vi "acquire single wave by LAN init subvi.vi"(0 "TCP Network Connection in":refnum<k5>, 11 "error in (no error)":errorcluster) -> (1 "CH1":string, 2 "Array 3":string[](array[string]), 3 "SEC/DIV":string, 4 "TCP Network Connection out":refnum<k5>, 6 "Array 2":string[](array[string]), 8 "Numeric":i32, 10 "data out":string, 13 "ID Query":string, 14 "Array":string[](array[string]), 15 "error out":errorcluster)   [LabVIEW 2013]
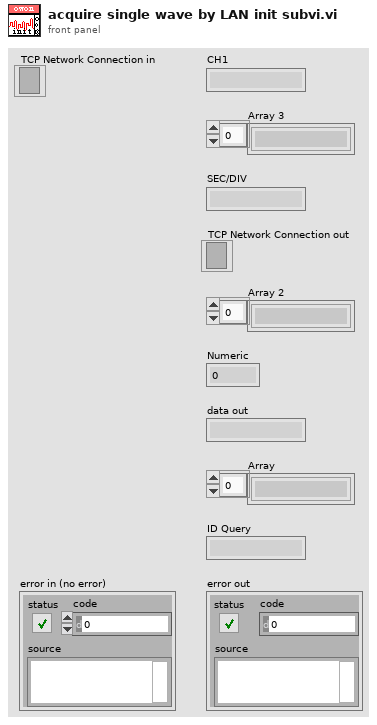
[diagram p1: front panel]
types:
  T1 = enum16{"Standard", "Buffered", "CRLF", "Immediate"}
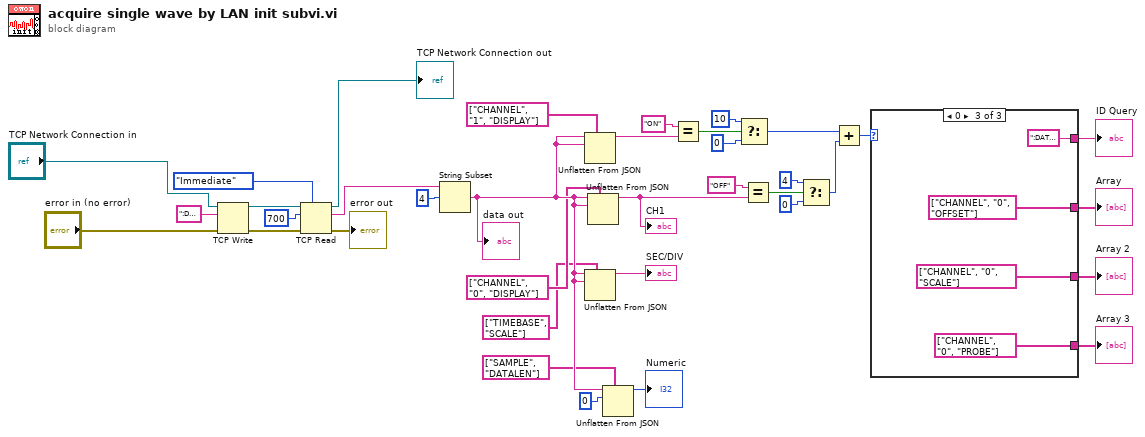
[diagram p0: block diagram]
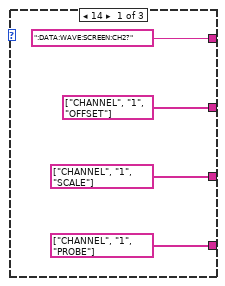
[diagram p2: hidden frame]
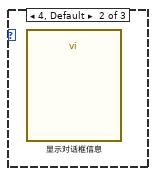
[diagram p3: hidden frame]
diagram:
  n1 = TCP Write(connection ID="TCP Network Connection in", data in=":DATA:WAVE:SCREEN:HEAD?" ("ID Query"), error in (no error)="error in (no error)") -> (connection ID out=w6:refnum<k5>, error out=w7:errorcluster)  [unwired: 1 in, 1 out]
  n2 = TCP Read(connection ID=w6, bytes to read=u32 700 ("byte count"), error in (no error)=w7, 7:T1."Immediate" ("mode (standard)")) -> (connection ID out=→"TCP Network Connection out":refnum<k5>, data out=w10:string, error out=→"error out":errorcluster)  [unwired: 1 in]
  n3 = String Subset(string=w10, offset (0)=4) -> (substring=w36:string)  [unwired: 1 in]
  "data out" <- w36
  n4 = Unflatten From JSON(path=string[] ["CHANNEL", "1", "DISPLAY"], JSON string=w36, type and defaults=w36) -> (value=w23:string)  [unwired: 4 in, 1 out]
  n5 = Unflatten From JSON(path=string[] ["TIMEBASE", "SCALE"], JSON string=w36, type and defaults=w36) -> (value=→"SEC/DIV":string)  [unwired: 4 in, 1 out]
  n6 = Unflatten From JSON(path=string[] ["CHANNEL", "0", "DISPLAY"], JSON string=w36, type and defaults=w36) -> (value=w29:string)  [unwired: 4 in, 1 out]
  "CH1" <- w29
  n7 = Unflatten From JSON(path=string[] ["SAMPLE", "DATALEN"], JSON string=w36, type and defaults=0) -> (value=→"Numeric":i32)  [unwired: 4 in, 1 out]
  n8 = Equal?(x="ON", y=w23) -> (x = y?=w25:bool)
  n9 = Select(t=10 ("offset (0)"), s=w25, f=0 ("offset (0)")) -> (s? t:f=w33:i32)
  n10 = Equal?(x="OFF", y=w29) -> (x = y?=w32:bool)
  n11 = Select(t=4 ("offset (0)"), s=w32, f=0 ("offset (0)")) -> (s? t:f=w34:i32)
  n12 = Add(x=w33, y=w34) -> (x+y=w35:i32)
  n13 = case shown="0" w35 {
    tunnel: [":DATA:WAVE:SCREEN:CH2?" ("ID Query") _ ":DATA:WAVE:SCREEN:CH1?" ("ID Query")] -> w19
    tunnel: [string[] ["CHANNEL", "1", "PROBE"] _ string[] ["CHANNEL", "0", "PROBE"]] -> w13
    tunnel: [string[] ["CHANNEL", "1", "SCALE"] _ string[] ["CHANNEL", "0", "SCALE"]] -> w14
    tunnel: [string[] ["CHANNEL", "1", "OFFSET"] _ string[] ["CHANNEL", "0", "OFFSET"]] -> w15
    frame 14 {
    }
    frame 4, Default {
      n14 = call "显示对话框信息"() -> ()  [unwired: 10 in, 2 out]
    }
    frame 0 {
    }
  }
  "ID Query" <- w19
  "Array" <- w15
  "Array 2" <- w14
  "Array 3" <- w13
